vi "FTW-Consumer-Destroy.vi"(0 "FTW-Consumer In":refnum<class "FTW-Consumer.lvclass">, 11 "error in":errorcluster) -> (15 "error out":errorcluster)   [LabVIEW 2013, in "FTW-Consumer.lvclass"]
uses:
  FTW-Consumer.lvclass
  FTW-Consumer.lvclass/FTW-Consumer.ctl
  Endpoint/FTW-Endpoint.lvclass
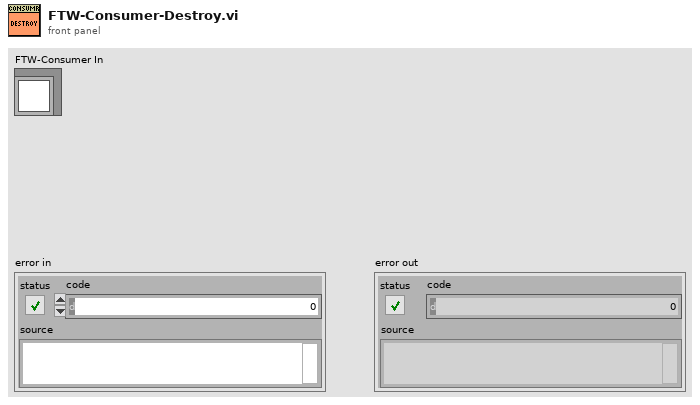
[diagram p1: front panel]
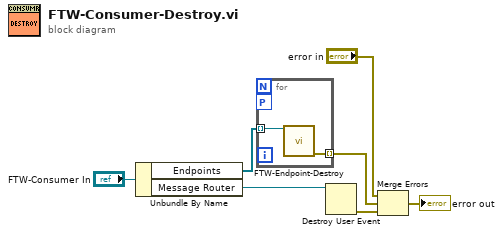
[diagram p0: block diagram]
diagram:
  n1 = Unbundle By Name("FTW-Consumer In") -> ("Endpoints"=w1:refnum<class "FTW-Endpoint.lvclass">[], "Message Router"=w4:refnum<user-event>)
  n2 = for {
    tunnel: [w9] -> w3 mode=indexing
    tunnel: w1 -> [w8] mode=indexing
    workers-P: _ -> [_]
    n3 = call-dynamic "FTW-Endpoint-Destroy.vi"("FTW Endpoint"=w8) -> ("error out"=w9:errorcluster)  [unwired: 14 in]
  }
  n4 = Destroy User Event(user event=w4) -> (error out=w2:errorcluster)  [unwired: 1 in]
  n5 = Merge Errors("error in", w3, w2) -> (→"error out":errorcluster)
